vi "RH_FGEN_WriteWfm.vi"(7 "FGEN Parameters":T1 {"Trigger Mode" items=["Single", "Continuous", "Stepped", "Burst"]}, 8 "error IO":errorcluster, 9 "Wfm Type":enum16{"Chirp", "MultiSine", "Sine"}(ring), 10 "Channel Name":string, 11 "FGEN Session In":refnum<k15>) -> (0 "error out":errorcluster, 3 "FGEN Session Out":refnum<k15>)   [LabVIEW 2023, in "ResourceHandling.lvlib"]
doc: "Generate Sine, Multi Sine or Chirp waveform"
uses:
  ResourceHandling.lvlib
  TypeDefs/RH_FGEN_Parameters.ctl
  <instrlib>/niFgen/niFgen.llb/niFgen Trigger Mode.ctl
  <instrlib>/niFgen/niFgen.llb/niFgen Write Waveform.vi
  <vilib>/Analysis/NI_AALBase.lvlib
panel:
  out "Normalized":dbl[](graph)
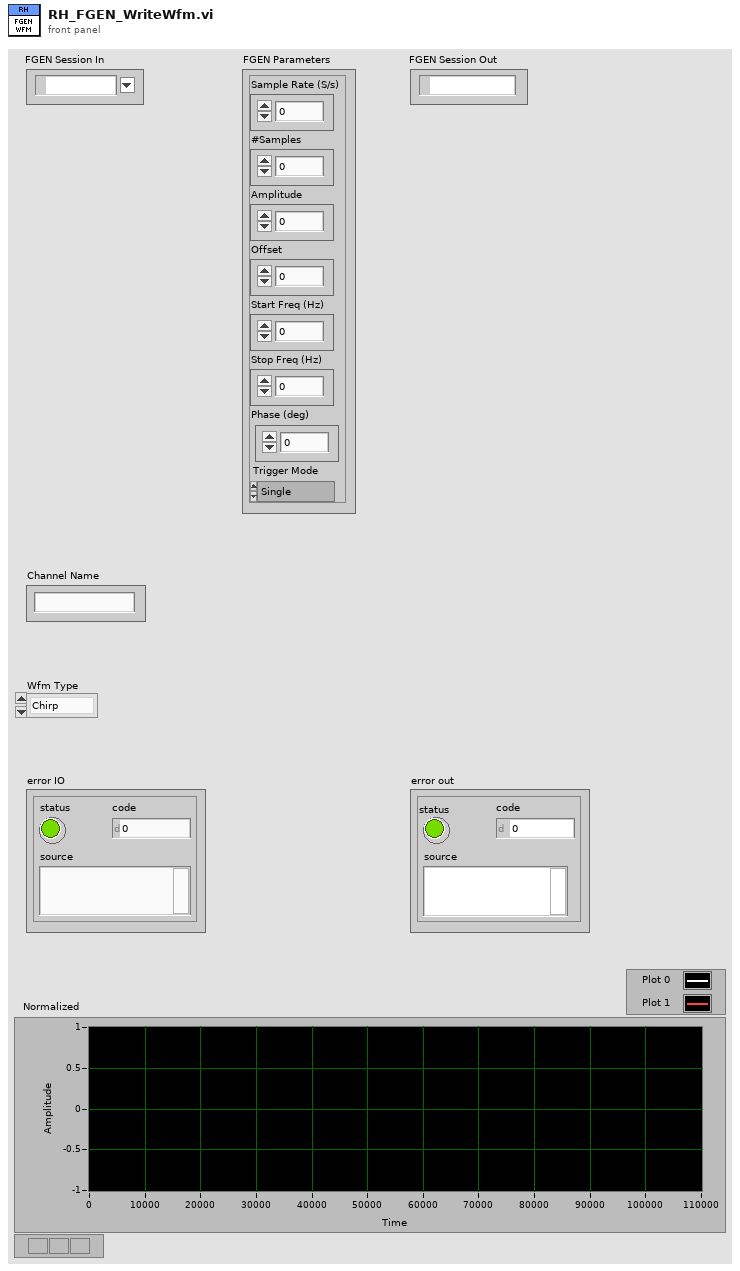
[diagram p1: front panel]
types:
  T1 = typedef "ResourceHandling.lvlib/RH_FGEN_Parameters.ctl" = cluster{"Sample Rate (S/s)":dbl, "#Samples":i32, "Amplitude":dbl, "Offset":dbl, "Start Freq (Hz)":dbl, "Stop Freq (Hz)":dbl, "Phase (deg)":dbl, "Trigger Mode":T2}
  T2 = typedef "niFgen Trigger Mode.ctl" = i32
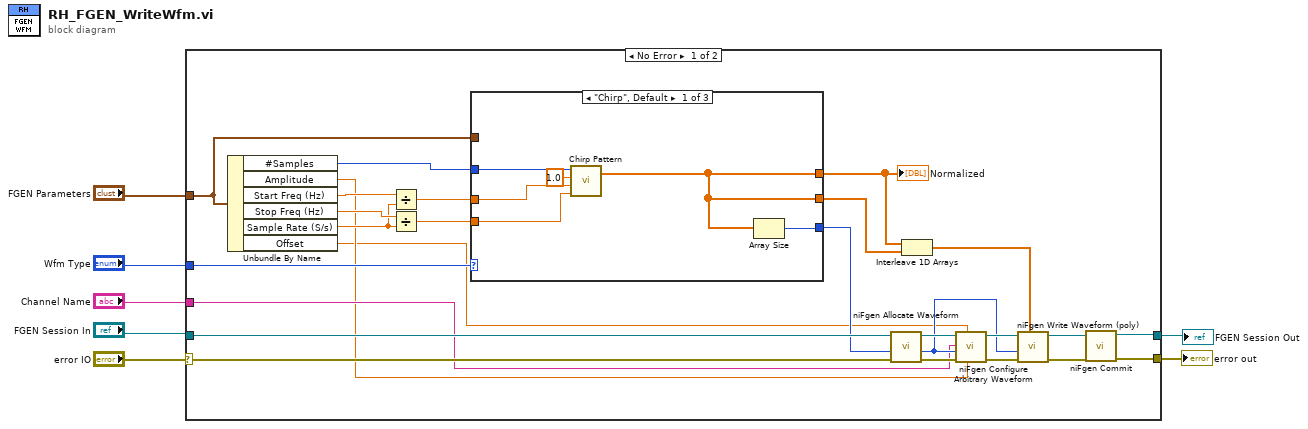
[diagram p0: block diagram]
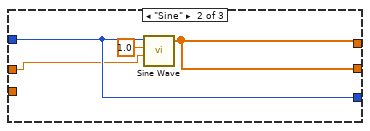
[diagram p2: hidden frame]
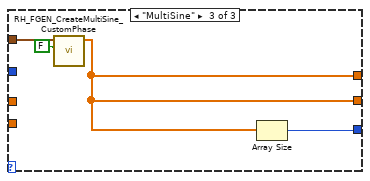
[diagram p3: hidden frame]
diagram:
  n1 = case shown="No Error" "error IO" {
    selector: "error IO" -> [w33 w49]
    tunnel: [w15 w49] -> w7
    tunnel: "FGEN Parameters" -> [w32 _]
    tunnel: "Wfm Type" -> [w31 _]
    tunnel: "FGEN Session In" -> [w21 w48]
    tunnel: "Channel Name" -> [w18 _]
    tunnel: [w14 w48] -> w1
    frame No Error {
      n2 = Unbundle By Name(w32) -> ("#Samples"=w29:i32, "Amplitude"=w11:dbl, "Start Freq (Hz)"=w20:dbl, "Stop Freq (Hz)"=w30:dbl, "Sample Rate (S/s)"=w13:dbl, "Offset"=w8:dbl)
      n3 = Divide(x=w20, y=w13) -> (x/y=w28:dbl)
      n4 = Divide(x=w30, y=w13) -> (x/y=w27:dbl)
      n5 = case shown="\"Chirp\", Default" w31 {
        tunnel: w29 -> [w37 w42 _]
        tunnel: w28 -> [w39 w40 _]
        tunnel: w27 -> [w38 _ _]
        tunnel: w32 -> [_ _ w46]
        tunnel: [w34 w42 w45] -> w19
        tunnel: [w35 w43 w44] -> w9
        tunnel: [w35 w43 w44] -> w10
        frame "Chirp", Default {
          n6 = call <vilib>:"Chirp Pattern.vi"("f2"=w38, "f1"=w39, "amplitude"=1.0, "samples"=w37) -> ("Chirp Pattern"=w35:dbl[])  [unwired: 1 out]
          n7 = Array Size(array=w35) -> (size(s)=w34:i32)
        }
        frame "Sine" {
          n8 = call <vilib>:"Sine Wave.vi"("samples"=w42, "amplitude"=1.0, "frequency"=w40) -> ("sine wave"=w43:dbl[])  [unwired: 2 in, 2 out]
        }
        frame "MultiSine" {
          n9 = call "RH_FGEN_CreateMultiSine_CustomPhase.vi"("Phase 0"=FALSE, "FGEN Parameters"=w46) -> ("sine wave"=w44:dbl[])  [unwired: 8 in, 1 out]
          n10 = Array Size(array=w44) -> (size(s)=w45:i32)
        }
      }
      "Normalized" <- w9
      n11 = call <instrlib>:"niFgen Allocate Waveform.vi"("error in (no error)"=w33, "Waveform Size"=w19, "Instrument Handle"=w21) -> ("error out"=w26:errorcluster, "Waveform Handle Out"=w22:i32, "Instrument Handle Out"=w25:refnum<k15>)  [unwired: 6 in]
      n12 = Interleave 1D Arrays(w9, w10) -> (w12:dbl[])
      n13 = call <instrlib>:"niFgen Configure Arbitrary Waveform.vi"("Gain"=w11, "Offset"=w8, "error in (no error)"=w26, "Waveform Handle"=w22, "Channel Name"=w18, "Instrument Handle"=w25) -> ("error out"=w23:errorcluster, "Instrument Handle Out"=w24:refnum<k15>)  [unwired: 4 in]
      n14 = call-poly <instrlib>:"niFgen Write Waveform (poly).vi"("Waveform Data"=w12, "error in (no error)"=w23, "Waveform Handle"=w22, "Instrument Handle"=w24) -> ("error out"=w16:errorcluster, "Instrument Handle Out"=w17:refnum<k15>)  [unwired: 5 in, 1 out]
      n15 = call <instrlib>:"niFgen Commit.vi"("error in (no error)"=w16, "Instrument Handle"=w17) -> ("error out"=w15:errorcluster, "Instrument Handle Out"=w14:refnum<k15>)  [unwired: 8 in]
    }
    frame Error {
    }
  }
  "error out" <- w7
  "FGEN Session Out" <- w1
